vi "TaskControl Page.vi"(8 "?":errorcluster) -> ()   [LabVIEW 2023, in "Vires VTD System Explorer.lvlib"]
uses:
  Vires VTD System Explorer.lvlib
  <vilib>/NI VeriStand/Custom Device API/Custom Device Item Ref.ctl
  Shared/Network Settings.ctl
  Shared/Protocol.ctl
  Shared/Timedloop Settings.ctl
  <vilib>/NI VeriStand/Custom Device API/Custom Device API.lvlib
  Shared/Vires VTD Shared.lvlib
panel:
  in  "Tab Control":enum32{"NetWork Settings", "Timedloop Settings"}(tab)
  in  "Network Settings":T1={"IP adress"="", "RDB"={"Protocol"=enum."UDP", "Tx Port"=48191, "Rx Port"=48191, "Buffer Size"=204800, "Timeout"=10}, "SCP"={"Protocol"=enum."TCP", "Tx Port"=48191, "Rx Port"=48191, "Buffer Size"=204800, "Timeout"=10}}
  in  "Timed Loop Settings for TaskControl Loop":T3={"Period(ms)"=2, "Priority"=100, "Processor"=-2}
  in  "Header":cluster{"Section Name":string}={"Section Name"="Custom Device Item Settings"}
  in  "Description":string
  in  "Name":string
  in  "Node Ptr":T4 format="%.0x"
  out "error out":errorcluster
  in  "SHDocVw.IWebBrowser2":refnum<k7>(container)
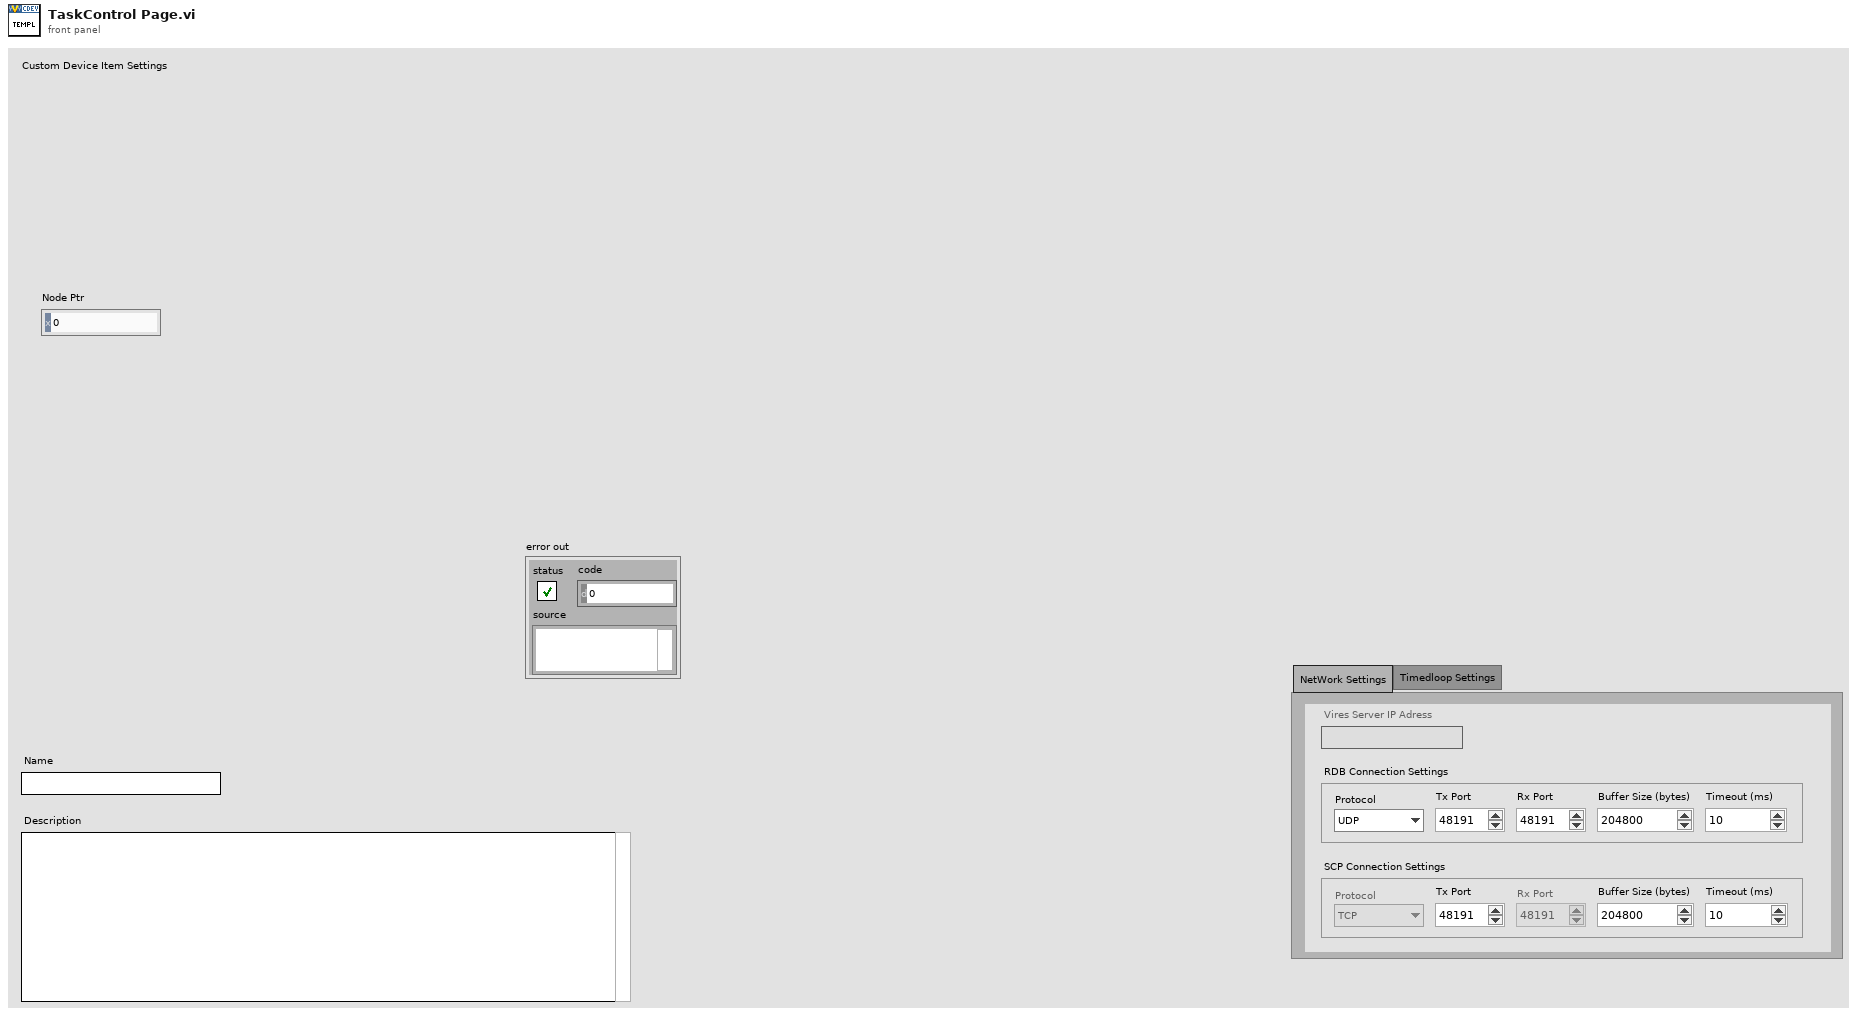
[diagram p1: front panel]
types:
  T1 = typedef "Vires VTD Shared.lvlib/Network Settings.ctl" = cluster{"IP adress":string, "RDB":cluster{"Protocol":T2, "Tx Port":u16, "Rx Port":u16, "Buffer Size":i32, "Timeout":u16}, "SCP":cluster{"Protocol":T2, "Tx Port":u16, "Rx Port":u16, "Buffer Size":i32, "Timeout":u16}}
  T2 = typedef "Vires VTD Shared.lvlib/Protocol.ctl" = enum16{"UDP", "TCP"}
  T3 = typedef "Vires VTD Shared.lvlib/Timedloop Settings.ctl" = cluster{"Period(ms)":i64, "Priority":i32, "Processor":i32}
  T4 = typedef "Custom Device API.lvlib/Custom Device Item Ref.ctl" = u64
  T5 = enum8{"Enabled", "Disabled", "Disabled and Grayed Out"}
  T6 = typedef "Custom Device API.lvlib/Custom Device Item Info.ctl" = cluster{"Name":string, "Is Channel":bool, "GUID":string, "Is Waveform":bool}
  T7 = typedef "Custom Device API.lvlib/Custom Device Commands.ctl" = enum16{"Default", "Item renamed", "Shutdown", "Dynamic button pressed"}
  T8 = cluster{"Protocol":T2, "Tx Port":u16, "Rx Port":u16, "Buffer Size":i32, "Timeout":u16}
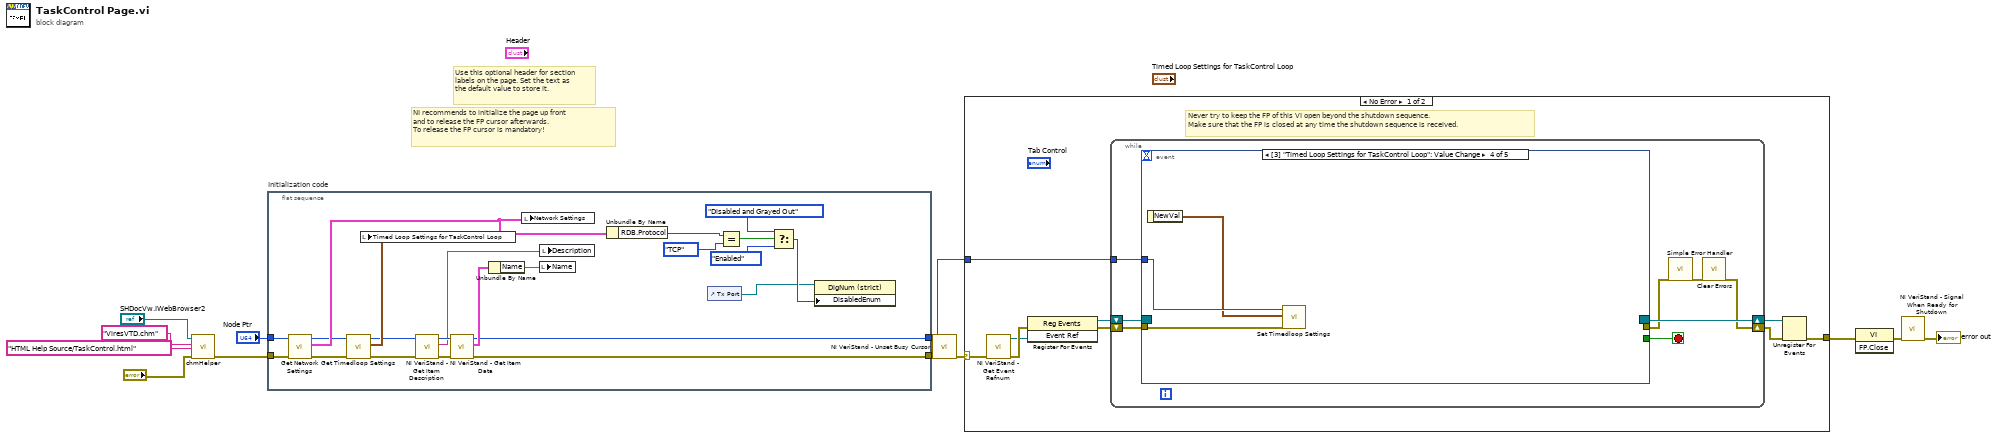
[diagram p0: block diagram]
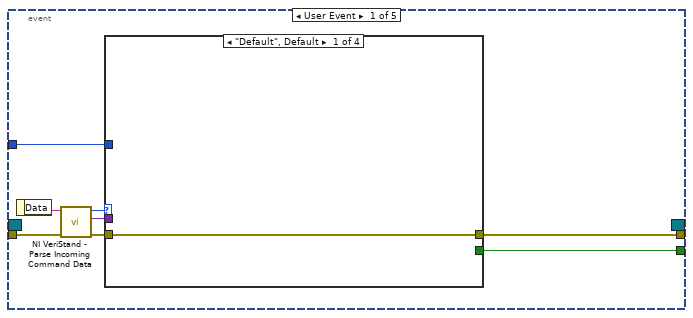
[diagram p2: hidden frame]
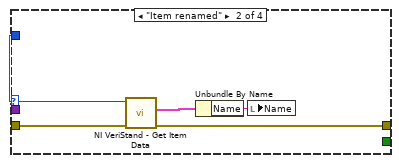
[diagram p3: hidden frame]
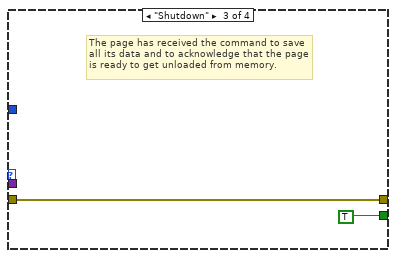
[diagram p4: hidden frame]
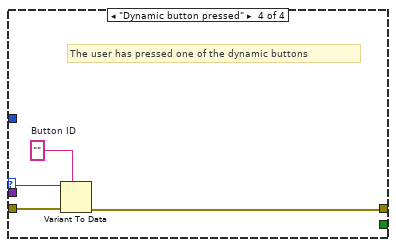
[diagram p5: hidden frame]
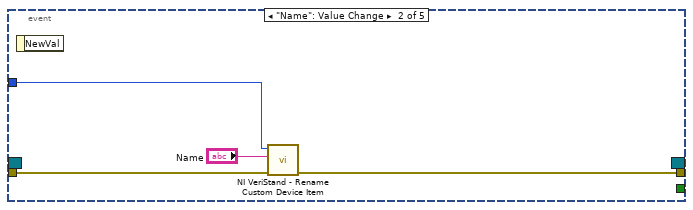
[diagram p6: hidden frame]
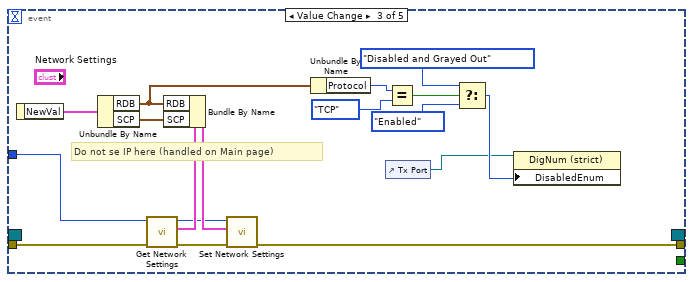
[diagram p7: hidden frame]
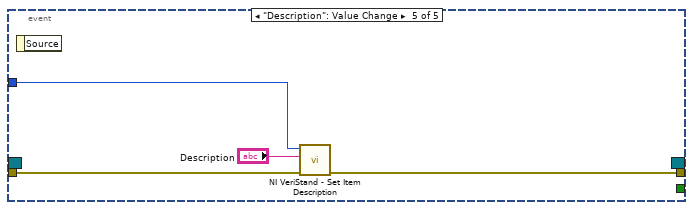
[diagram p8: hidden frame]
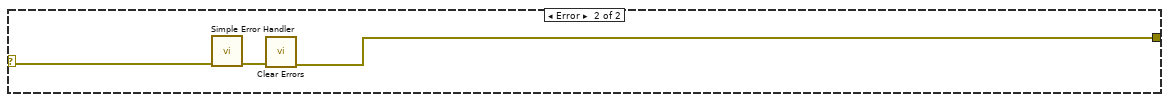
[diagram p9: hidden frame]
diagram:
  # "Use this optional header for section labels on the page. Set the text as the default value to store it."
  # "NI recommends to initialize the page up front\nand to release the FP cursor afterwards.\nTo release the FP cursor is mandatory!"
  n1 = call "chmHelper.vi"("error in (no error)"="?", "HTML File"="HTML Help Source/TaskControl.html", "Main CHM File"="ViresVTD.chm" ("HTML File"), "Automation Refnum in"="SHDocVw.IWebBrowser2") -> ("error out"=w2:errorcluster)  [unwired: 7 in]
  n2 = flat-sequence "Initialization code" {
    tunnel: "Node Ptr" -> [w28]
    tunnel: [w29] -> w8
    tunnel: w2 -> [w27]
    tunnel: [w26] -> w1
    frame #0 {
      n3 = call "Get Network Settings.vi"("error in"=w27, "Item Ref in"=w28) -> ("error out"=w14:errorcluster, "Network Settings"=w25:T1, "Item Ref out"=w16:T4)  [unwired: 7 in]
      n4 = call "Get Timedloop Settings.vi"("error in"=w14, "Item Ref in"=w16) -> ("error out"=w13:errorcluster, "Timed Loop Settings"=w17:T3, "Item Ref out"=w15:T4)  [unwired: 7 in]
      n5 = local write "Timed Loop Settings for TaskControl Loop"(w17) -> ()
      n6 = call <vilib>:"NI VeriStand - Get Item Description.vi"("error in (no error)"=w13, "Item Ref in"=w15) -> ("error out"=w32:errorcluster, "Description"=w33:string, "Item Ref out"=w34:T4)  [unwired: 7 out]
      n7 = call <vilib>:"NI VeriStand - Get Item Data.vi"("error in (no error)"=w32, "Item Ref in"=w34) -> ("error out"=w26:errorcluster, "Item Info"=w31:T6, "Item Ref out"=w29:T4)  [unwired: 7 out]
      n8 = Unbundle By Name(w31) -> ("Name"=w30:string)
      n9 = local write "Network Settings"(w25) -> ()
      n10 = local write "Name"(w30) -> ()
      n11 = local write "Description"(w33) -> ()
      n12 = Unbundle By Name(w25) -> ("RDB.Protocol"=w19:T2)
      n13 = control-ref of="Tx Port"() -> (w18:refnum<vi>)
      n14 = Equal?(x=w19, y=Protocol."TCP") -> (x = y?=w23:bool)
      n15 = Select(t=T5."Disabled and Grayed Out" ("Disabled"), s=w23, f=T5."Enabled" ("Disabled")) -> (s? t:f=w22:T5)
      n16 = property class="DigNum (strict)"(reference=w18, "DisabledEnum"=w22) -> ()  [unwired: 1 in, 2 out]
    }
  }
  n17 = call <vilib>:"NI VeriStand - Unset Busy Cursor.vi"("error in (no error)"=w1) -> ("error out"=w9:errorcluster)  [unwired: 10 out]
  n18 = case shown="No Error" w9 {
    selector: w9 -> [w35 w102]
    tunnel: [w40 w100] -> w12
    tunnel: w8 -> [w36 _]
    frame No Error {
      # "Never try to keep the FP of this VI open beyond the shutdown sequence.\nMake sure that the FP is closed at any time the shutdown sequence is received."
      n19 = call <vilib>:"NI VeriStand - Get Event Refnum.vi"("error in (no error)"=w35) -> ("error out"=w43:errorcluster, "Event Ref"=w39:refnum<user-event>)  [unwired: 9 out]
      n20 = register-events(error in=w43, w39) -> (reference out=w37:refnum<event-registration>, error out=w38:errorcluster)  [unwired: 1 in]
      n21 = while {
        tunnel: w36 -> [w47]
        shift-right: [w44] -> w41
        shift-left: w38 -> [w50]
        shift-right: [w51] -> w42
        shift-left: w37 -> [w49]
        stop <- w48 stop-if-true
        n22 = event shown="[3] \"Timed Loop Settings for TaskControl Loop\": Value Change" {
          selector: w49 -> [_ _ _ _ _]
          dyn-events: [_ _ _ _ _] -> w51
          timeout: _ -> [_ _ _ _ _]
          tunnel: w50 -> [w59 w75 w89 w94 w98]
          tunnel: [w55 _ _ _ _] -> w48
          tunnel: [w54 w74 w88 _ w97] -> w46
          tunnel: w47 -> [w53 w73 w87 w95 w99]
          event User Event {
            n23 = event-data() -> ("Data"=w58:string)  [unwired: 1 out]
            n24 = call <vilib>:"NI VeriStand - Parse Incoming Command Data.vi"("error in (no error)"=w59, "Incoming data"=w58) -> ("error out"=w57:errorcluster, "Outgoing data"=w52:variant, "Action"=w56:T7)  [unwired: 7 out]
            n25 = case shown="\"Default\", Default" w56 {
              tunnel: w57 -> [w60 w65 w66 w71]
              tunnel: [_ _ TRUE _] -> w55
              tunnel: [w60 w63 w66 w68] -> w54
              tunnel: w53 -> [_ w61 _ _]
              tunnel: w52 -> [_ _ _ w70]
              frame "Default", Default {
              }
              frame "Item renamed" {
                n26 = call <vilib>:"NI VeriStand - Get Item Data.vi"("error in (no error)"=w65, "Item Ref in"=w61) -> ("error out"=w63:errorcluster, "Item Info"=w64:T6)  [unwired: 8 out]
                n27 = Unbundle By Name(w64) -> ("Name"=w62:string)
                n28 = local write "Name"(w62) -> ()
              }
              frame "Shutdown" {
                # "The page has received the command to save all its data and to acknowledge that the page is ready to get unloaded from memory."
              }
              frame "Dynamic button pressed" {
                w69 = ""  # Button ID
                # "The user has pressed one of the dynamic buttons"
                n29 = Variant To Data(error in=w71, type=w69, Variant=w70) -> (error out=w68:errorcluster)  [unwired: 1 out]
              }
            }
          }
          event "Name": Value Change {
            n30 = event-data() -> ()  [unwired: 2 out]
            n31 = call <vilib>:"NI VeriStand - Rename Custom Device Item.vi"("error in (no error)"=w75, "New Name"="Name", "Item Ref in"=w73) -> ("error out"=w74:errorcluster)  [unwired: 1 in, 7 out]
          }
          event Value Change {
            # "Do not se IP here (handled on Main page)"
            n32 = event-data() -> ("NewVal"=w86:T1)  [unwired: 1 out]
            n33 = Unbundle By Name(w86) -> ("RDB"=w83:T8, "SCP"=w85:T8)
            n34 = call "Get Network Settings.vi"("error in"=w89, "Item Ref in"=w87) -> ("error out"=w84:errorcluster, "Network Settings"=w91:T1, "Item Ref out"=w90:T4)  [unwired: 7 in]
            n35 = Bundle By Name(cluster=w91, "RDB"=w83, "SCP"=w85) -> (w92:T1)
            n36 = call "Set Network Settings.vi"("error in"=w84, "Network Settings"=w92, "Item Ref in"=w90) -> ("error out"=w88:errorcluster)  [unwired: 7 in, 1 out]
            n37 = Unbundle By Name(w83) -> ("Protocol"=w82:T2)
            n38 = control-ref of="Tx Port"() -> (w76:refnum<vi>)
            n39 = Equal?(x=w82, y=Protocol."TCP") -> (x = y?=w80:bool)
            n40 = Select(t=T5."Disabled and Grayed Out" ("Disabled"), s=w80, f=T5."Enabled" ("Disabled")) -> (s? t:f=w79:T5)
            n41 = property class="DigNum (strict)"(reference=w76, "DisabledEnum"=w79) -> ()  [unwired: 1 in, 2 out]
          }
          event Value Change {
            n42 = event-data() -> ("NewVal"=w93:T3)  [unwired: 1 out]
            n43 = call "Set Timedloop Settings.vi"("error in"=w94, "Timed Loop Settings"=w93, "Item Ref in"=w95) -> ()  [unwired: 7 in, 2 out]
          }
          event "Description": Value Change {
            n44 = event-data() -> ()  [unwired: 2 out]
            n45 = call <vilib>:"NI VeriStand - Set Item Description.vi"("error in (no error)"=w98, "Description"="Description", "Item Ref in"=w99) -> ("error out"=w97:errorcluster)  [unwired: 8 out]
          }
        }
        n46 = call <vilib>:"Simple Error Handler.vi"("error in (no error)"=w46) -> ("error out"=w45:errorcluster)  [unwired: 1 in, 7 out]
        n47 = call <vilib>:"Clear Errors.vi"("error in (no error)"=w45) -> ("error out"=w44:errorcluster)  [unwired: 1 in, 5 out]
      }
      n48 = Unregister For Events(event registration refnum=w42, error in=w41) -> (error out=w40:errorcluster)
    }
    frame Error {
      n49 = call <vilib>:"Simple Error Handler.vi"("error in (no error)"=w102) -> ("error out"=w101:errorcluster)  [unwired: 1 in, 7 out]
      n50 = call <vilib>:"Clear Errors.vi"("error in (no error)"=w101) -> ("error out"=w100:errorcluster)  [unwired: 1 in, 5 out]
    }
  }
  n51 = invoke class="VI" method="FP.Close"(error in=w12) -> (error out=w11:errorcluster)  [unwired: 2 in, 2 out]
  n52 = call <vilib>:"NI VeriStand - Signal When Ready for Shutdown.vi"("error in (no error)"=w11) -> ("error out"=→"error out":errorcluster)  [unwired: 10 out]
